vi "interfaceLoop tabStateCheck.vi"(8 "error in (no error)":errorcluster, 9 "connectStateRefnum":refnum<data-value>, 11 "Stop":refnum<vi>) -> (0 "error out":errorcluster)   [LabVIEW 2018]
uses:
  <vilib>/Platform/TimedLoop/XDataNode/timing_clust.ctl
  <vilib>/Platform/TimedLoop/XDataNode/nitl_modes.ctl
  <vilib>/Platform/TimedLoop/XDataNode/wakeup.ctl
  <vilib>/Platform/TimedLoop/XDataNode/XDataNode.xnode
  <vilib>/Platform/TimedLoop/XDataNode/XDNodeRunTimeDep.lvlib
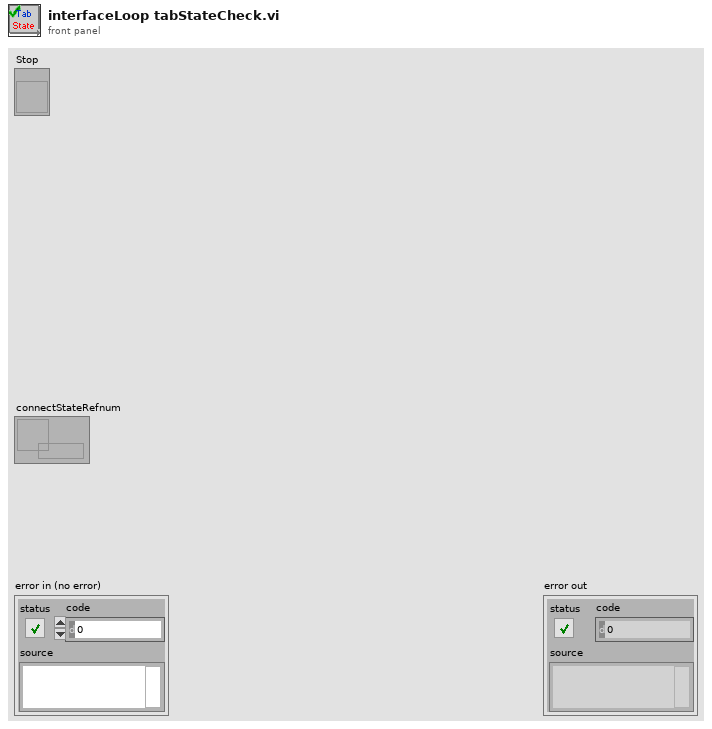
[diagram p1: front panel]
types:
  T1 = typedef "XDNodeRunTimeDep.lvlib/timing_clust.ctl" = cluster{"Expected End [f-1]":u64, "Actual End [f-1]":u64, "Finished Late? [f-1]":bool, "Expected End [i-1]":u64, "Actual End [i-1]":u64, "Finished Late? [i-1]":bool, "Expected Start [i]":u64, "Actual Start [i]":u64, "Expected Start [f]":u64, "Actual Start [f]":u64, "Source Name":string, "Structure Name":string, "Period":i64, "Deadline":i64, "Offset":i64, "Start":i64, "Priority":i32, "Timeout":i32, "Mode":T2, "Wakeup Reason":T3, "Error":errorcluster, "Source Type":string, "Secondary Source Type":string, "Global End Time":u64, "Global Start Time":u64, "Frame Duration":u64, "Iteration Duration":u64, "Assigned CPU":i32, "I/O Scan Engine Mode":u32}
  T2 = typedef "XDNodeRunTimeDep.lvlib/nitl_modes.ctl" = enum32{"No Change", "Process missed periods, maintain original phase", "Discard missed periods, maintain original phase", "Process missed periods, ignore original phase", "Discard missed periods, ignore original phase"}
  T3 = typedef "XDNodeRunTimeDep.lvlib/wakeup.ctl" = enum32{"Normal", "Aborted", "Asynchronous wakeup", "Timing source error", "Timed loop error", "Timeout"}
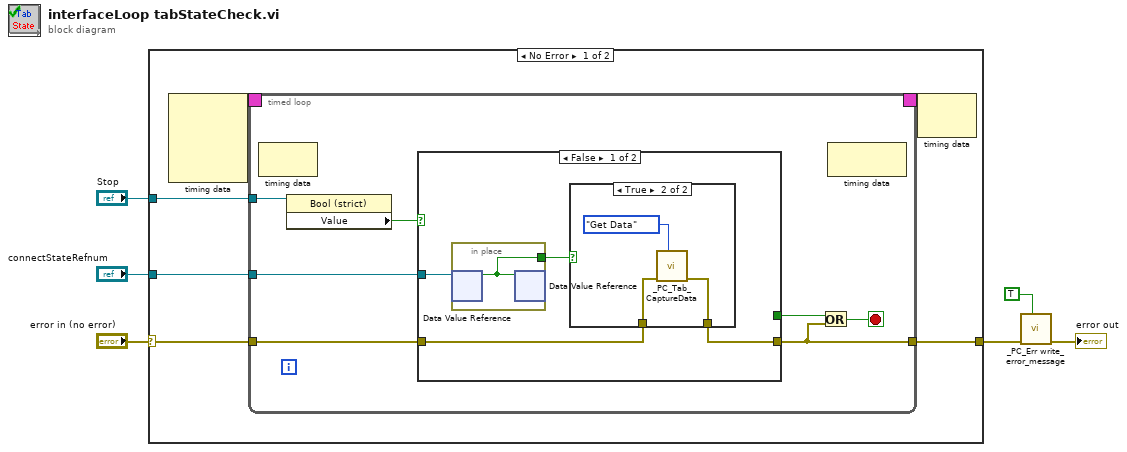
[diagram p0: block diagram]
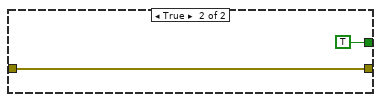
[diagram p3: hidden frame]
diagram:
  n1 = case shown="No Error" "error in (no error)" {
    selector: "error in (no error)" -> [w10 w35]
    tunnel: [w9 w35] -> w2
    tunnel: "Stop" -> [w12 _]
    tunnel: "connectStateRefnum" -> [w11 _]
    frame No Error {
      n2 = node-c288() -> (w8:T1)  [unwired: 4 in]
      n3 = timed-loop {
        tunnel: w12 -> [w19]
        tunnel: w11 -> [w17]
        tunnel: w10 -> [w16]
        tunnel: [w13] -> w9
        timing: w8 -> [_]
        timing-out: [_] -> w7
        stop <- w14 stop-if-true
        n4 = node-c288() -> ()  [unwired: 1 in, 1 out]
        n5 = property class="Bool (strict)"(reference=w19) -> ("Value"=w18:bool)  [unwired: 1 in, 2 out]
        n6 = case shown="False" w18 {
          tunnel: w17 -> [w25 _]
          tunnel: w16 -> [w23 w32]
          tunnel: [w22 w32] -> w13
          tunnel: [_ TRUE] -> w15
          frame False {
            n7 = in-place {
              in-place-border: [w30] -> w24
              n8 = in-place-dvr #1(w25) -> (w30:bool)  [unwired: 1 out]
              n9 = in-place-dvr #1(w30) -> ()  [unwired: 2 out]
            }
            n10 = case shown="True" w24 {
              tunnel: w23 -> [w26 w29]
              tunnel: [w26 w28] -> w22
              frame False {
              }
              frame True {
                n11 = call "_PC_Tab_CaptureData.vi"("Function"=enum16{"Init", "Get Data", "Update", "Close"}."Get Data", "error in (no error)"=w29) -> ("error out"=w28:errorcluster)  [unwired: 9 in]
              }
            }
          }
          frame True {
          }
        }
        n12 = Or(x=w15, y=w13) -> (x .or. y?=w14:bool)
        n13 = node-c288() -> ()  [unwired: 1 in, 1 out]
      }
      n14 = node-c288(w7) -> ()  [unwired: 1 out]
    }
    frame Error {
    }
  }
  n15 = call "_PC_Err write_error_message.vi"("show msg( T )"=TRUE, "error in"=w2) -> ("error out"=→"error out":errorcluster)  [unwired: 9 in]
